vi "Terminate.vi"(8 "error in (no error)":errorcluster, 10 "Message in":refnum<class "TerminateMessage.lvclass">, 11 "ConfocalStage in":refnum<class "ConfocalStage.lvclass">) -> (0 "error out":errorcluster, 3 "ConfocalStage out":refnum<class "ConfocalStage.lvclass">)   [LabVIEW 2012, in "ConfocalStage.lvclass"]
doc: "This member function is called when the statemachine in the run.vi receives an 'terminate' command. It closes the RabbitMQ connection. \n\nOverride this member function in your derived class to release all previously acquired resources (but don't forget to call the parent method). If your component has subcomponents, they count as resources, and you have to release them by calling their own terminate functions."
uses:
  ConfocalStage.lvclass
  <vilib>/Distrio/Murmex/TerminateMessage/TerminateMessage.lvclass
  <vilib>/Distrio/Murmex/Murmex/Murmex.lvclass
panel:
  # "This method is called when the TERMINATE\ntrigger is sent. \n\nOverride this method when your component needs to\nrespond to this trigger. \n\nCall parent for proper implementation"
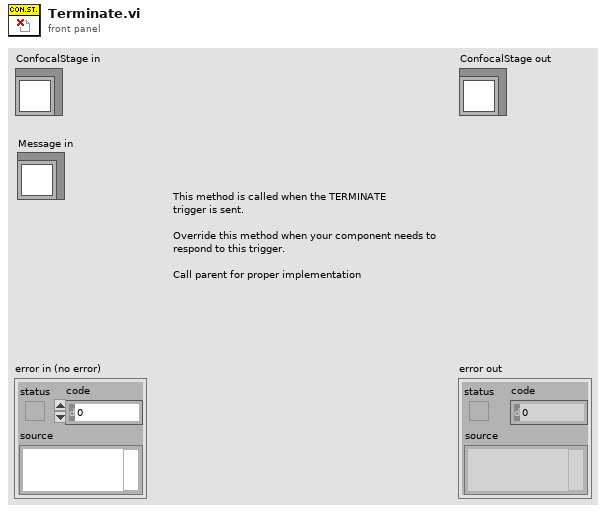
[diagram p1: front panel]
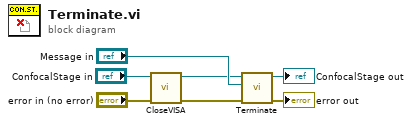
[diagram p0: block diagram]
diagram:
  n1 = call-dynamic "CloseVISA.vi"("error in (no error)"="error in (no error)", "ConfocalStage in"="ConfocalStage in") -> ("error out"=w1:errorcluster, "ConfocalStage out"=w3:refnum<class "ConfocalStage.lvclass">)  [unwired: 8 in]
  n2 = call-parent "Terminate.vi"("error in (no error)"=w1, "Message in"="Message in", "Murmex in"=w3) -> ("error out"=→"error out":errorcluster, "Murmex out"=→"ConfocalStage out":refnum<class "ConfocalStage.lvclass">)  [unwired: 7 in]
